vi "zakres wprowadzanego pixela do 1400 pixeli od startu.vi"(10 "Numeric 2":i32, 11 "Numeric":i32) -> (3 "Boolean":bool)   [LabVIEW 2015, in "Biblioteka moduł map v3.lvlib" / "Pomocnicze.lvlib"]
uses:
  Pomocnicze.lvlib
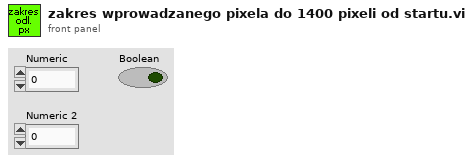
[diagram p1: front panel]
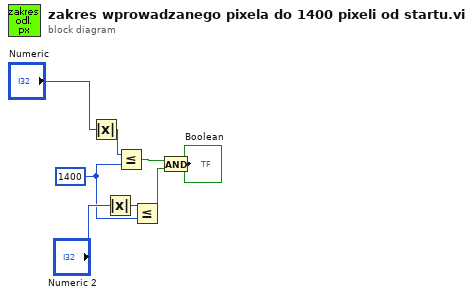
[diagram p0: block diagram]
diagram:
  w3 = 1400 ("y")
  n1 = Absolute Value(x="Numeric") -> (abs(x)=w7:i32)
  n2 = Absolute Value(x="Numeric 2") -> (abs(x)=w5:i32)
  n3 = Less Or Equal?(x=w7, y=w3) -> (x <= y?=w1:bool)
  n4 = Less Or Equal?(x=w5, y=w3) -> (x <= y?=w2:bool)
  n5 = And(x=w1, y=w2) -> (x .and. y?=→"Boolean":bool)
